vi "ZCR_IN_SIN_0_finder.vi"(10 "Noise amplitude":dbl format="%.2p", 11 "ZCR ON":waveform(dbl)[](array[waveform])=[{"t0"=timestamp(3707890383.8976955 s since 1904-01-01), "dt"=9.999999999999999e-05, "Y"=array[20000 elements], "attributes"=variant("NI_ChannelName"=variant(string "Tension_0"), "NI_UnitDescription"=variant(string "Volts"))}, {"t0"=timestamp(3707890383.8977456 s since 1904-01-01), "dt"=9.999999999999999e-05, "Y"=array[20000 elements], "attributes"=variant("NI_ChannelName"=variant(string "Tension_1"), "NI_UnitDescription"=variant(string "Volts"))}]) -> (3 "OFF SIN":i32[](array[numeric]))   [LabVIEW 2020, in "Library Commun.lvlib" / "Nodon_ZCR.lvclass"]
uses:
  Nodon_ZCR.lvclass
  <vilib>/Utility/miscctls.llb/LVRangeTypeDef.ctl
  <vilib>/measure/matone.llb/Extract Single Tone Information 1 Chan.vi
  Nodon_ZCR.lvclass/Nodon_ZCR.ctl
  <vilib>/measure/NI_MABase.lvlib
  <vilib>/measure/NI_MAPro.lvlib
panel:
  out "Waveform Graph 3":waveform(dbl)[](graph)
  in  "Point 2":i32
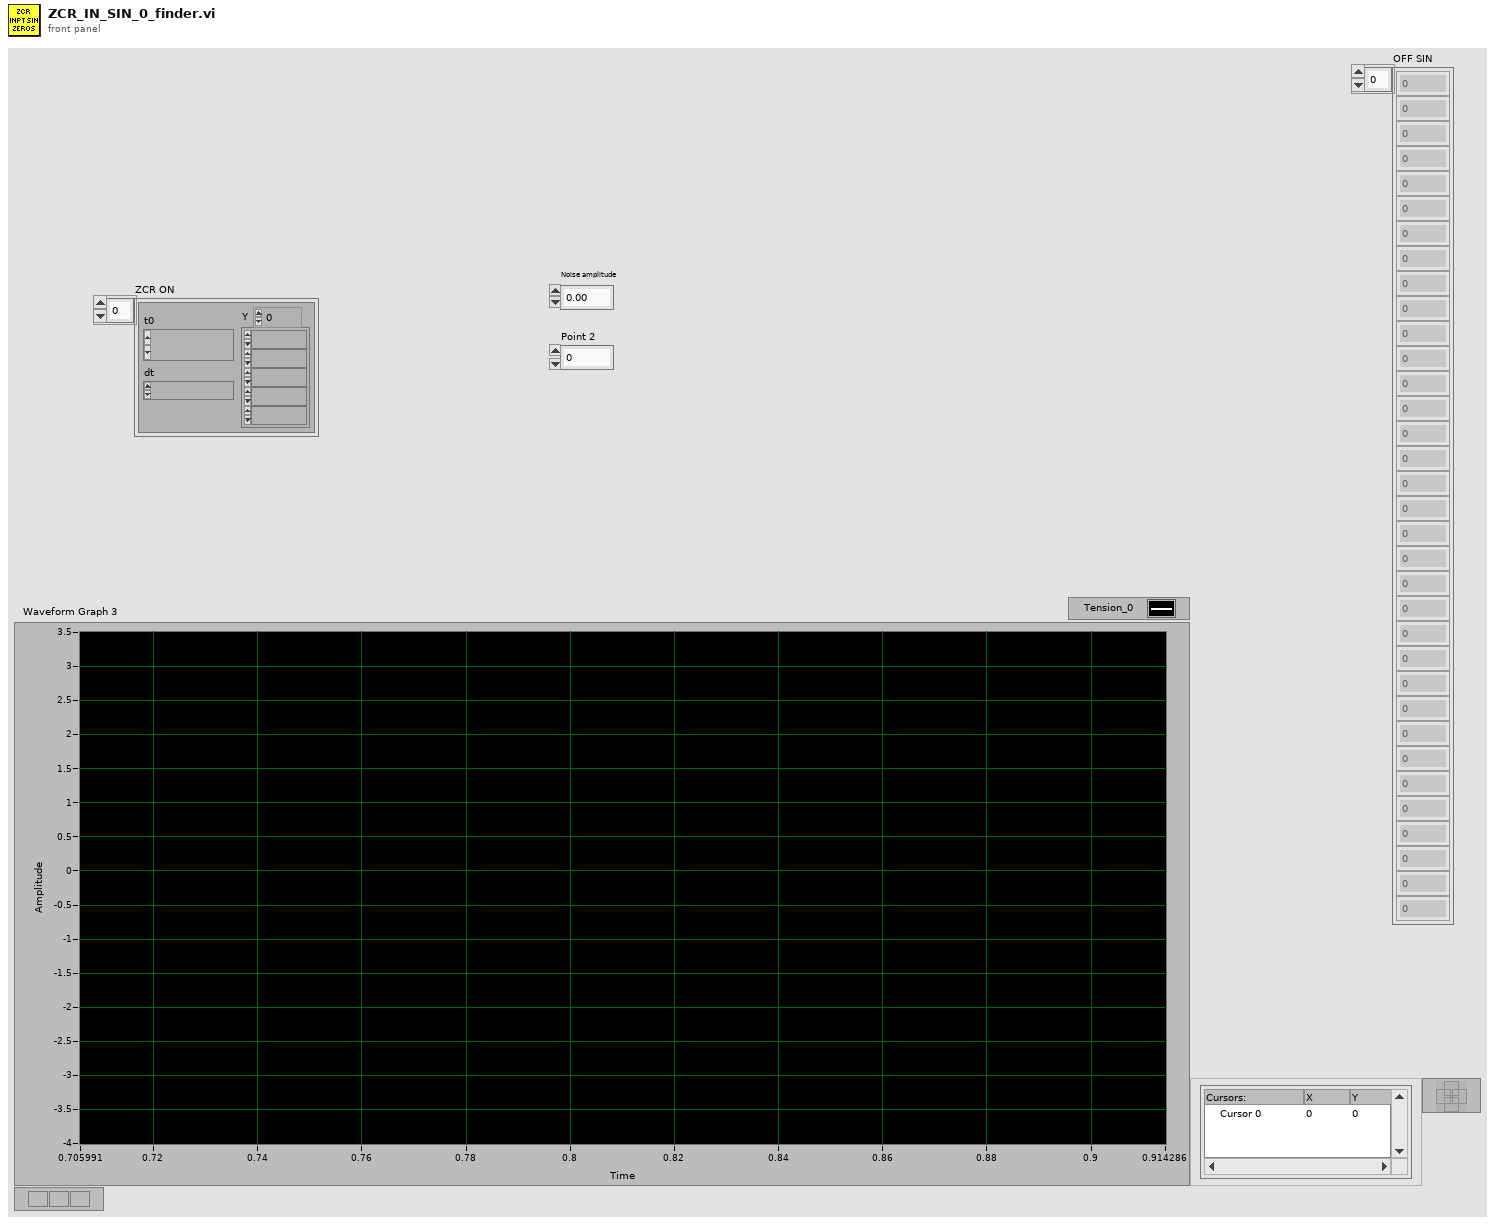
[diagram p1: front panel]
types:
  T1 = typedef "LVRangeTypeDef.ctl" = cluster{"Minimum":dbl, "Maximum":dbl, "Increment":dbl, "Minor Increment":dbl, "Start":dbl}
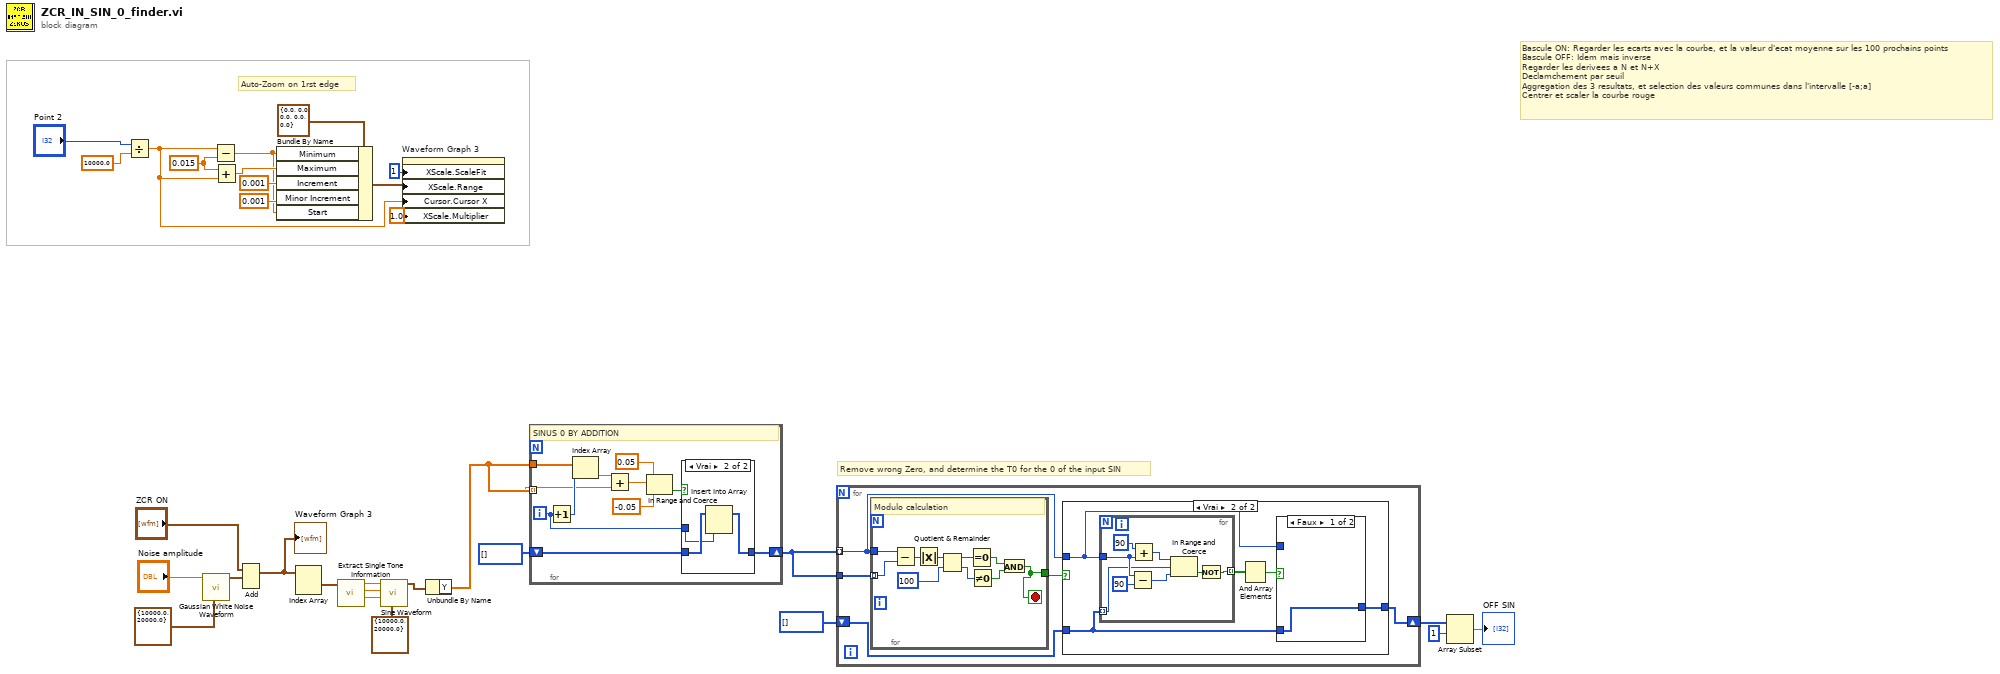
[diagram p0: block diagram]
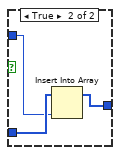
[diagram p3: hidden frame]
diagram:
  w20 = 0.015
  # "Bascule ON: Regarder les ecarts avec la courbe, et la valeur d'ecat moyenne sur les 100 prochains points\nBascule OFF: Idem mais inverse\nRegarder les derivees a N et N+X\nDeclamchement par seuil\nAggregation des 3 resultats, et selection des valeurs communes dans l'intervalle [-a;a]\nCentrer et scaler la courbe rouge"
  # "Remove wrong Zero, and determine the T0 for the 0 of the input SIN"
  # "Auto-Zoom on 1rst edge"
  n1 = Divide(x="Point 2", y=10000.0) -> (x/y=w11:dbl)
  n2 = call <vilib>:"Gaussian White Noise Waveform.vi"("sampling info"=cluster{"Fs":dbl, "#s":dbl} {"Fs"=10000.0, "#s"=20000.0}, "standard deviation"="Noise amplitude") -> ("signal out"=w27:waveform(dbl))  [unwired: 8 in, 1 out]
  n3 = Subtract(x=w11, y=w20) -> (x-y=w15:dbl)
  n4 = Add(x=w20, y=w11) -> (x+y=w18:dbl)
  n5 = Add(1:w27, 2:"ZCR ON") -> (0:w9:waveform(dbl)[])  [unwired: 1 in, 1 out]
  "Waveform Graph 3" <- w9
  n6 = Bundle By Name(cluster=T1 {"Minimum"=0.0, "Maximum"=0.0, "Increment"=0.0, "Minor Increment"=0.0, "Start"=0.0} ("X Scale.Range"), "Minimum"=w15, "Maximum"=w18, "Increment"=0.001, "Minor Increment"=0.001, "Start"=w15) -> (w14:T1)
  n7 = Index Array(array=w9) -> (element #1=w1:waveform(dbl))  [unwired: 2 in, 1 out]
  n8 = call-poly <vilib>:"Extract Single Tone Information.vi"("time signal in"=w1) -> ("detected phase (deg)"=w26:dbl, "detected amplitude"=w25:dbl, "detected frequency"=w24:dbl)  [unwired: 5 in, 3 out]
  n9 = call <vilib>:"Sine Waveform.vi"("sampling info"=cluster{"Fs":dbl, "#s":dbl} {"Fs"=10000.0, "#s"=20000.0}, "phase"=w26, "amplitude"=w25, "frequency"=w24) -> ("signal out"=w6:waveform(dbl))  [unwired: 6 in, 1 out]
  n10 = property on="Waveform Graph 3" class="GraphWF (strict)"("XScale.ScaleFit"=u8 1 ("X Scale.Scale Fit"), "XScale.Range"=w14, "Cursor.Cursor X"=w11, "XScale.Multiplier"=1.0 ("X Scale.Offset and Multiplier:Multiplier")) -> ()  [unwired: 2 in, 2 out]
  n11 = Unbundle By Name(w6) -> ("Y"=w5:dbl[])
  n12 = for {
    tunnel: w5 -> [w41]
    tunnel: w5 -> [w38] mode=indexing
    shift-right: [w36] -> w8
    shift-left: i32[] [] -> [w37]
    i -> [w35]
    # "SINUS 0 BY ADDITION"
    n13 = Increment(x=w35) -> (x+1=w40:i32)
    n14 = Index Array(array=w41, index=w40) -> (element=w39:dbl)
    n15 = Add(x=w39, y=w38) -> (x+y=w34:dbl)
    n16 = In Range and Coerce(upper limit=0.05 ("lower limit"), x=w34, lower limit=-0.05) -> (In Range?=w33:bool)  [unwired: 1 out]
    n17 = case shown="Vrai" w33 {
      tunnel: [w42 w44] -> w36
      tunnel: w37 -> [w42 w45]
      tunnel: w35 -> [_ w43]
      frame False {
      }
      frame True {
        n18 = Insert Into Array(array=w45, new element=w43) -> (w44:i32[])  [unwired: 1 in]
      }
    }
  }
  n19 = for {
    tunnel: w8 -> [w46] mode=indexing
    tunnel: w8 -> [w50]
    shift-right: [w47] -> w4
    shift-left: i32[] [] -> [w48]
    n20 = for {
      tunnel: w46 -> [w78]
      tunnel: w50 -> [w77] mode=indexing
      tunnel: [w69] -> w49
      stop <- w69 stop-if-true
      # "Modulo calculation"
      n21 = Subtract(x=w78, y=w77) -> (x-y=w76:i32)
      n22 = Absolute Value(x=w76) -> (abs(x)=w75:i32)
      n23 = Quotient & Remainder(x=w75, y=100) -> (x-y*floor(x/y)=w73:i32, floor(x/y)=w72:i32)
      n24 = Equal To 0?(x=w73) -> (x = 0?=w71:bool)
      n25 = Not Equal To 0?(x=w72) -> (x != 0?=w70:bool)
      n26 = And(x=w71, y=w70) -> (x .and. y?=w69:bool)
    }
    n27 = case shown="Vrai" w49 {
      tunnel: w48 -> [w51 w54]
      tunnel: [w51 w53] -> w47
      tunnel: w46 -> [_ w52]
      frame False {
      }
      frame True {
        n28 = for {
          tunnel: w52 -> [w64]
          tunnel: w54 -> [w61] mode=indexing
          tunnel: [w62] -> w56 mode=indexing
          n29 = Subtract(x=w64, y=90) -> (x-y=w65:i32)
          n30 = Add(x=90, y=w64) -> (x+y=w66:i32)
          n31 = In Range and Coerce(upper limit=w66, x=w61, lower limit=w65) -> (In Range?=w63:bool)  [unwired: 1 out]
          n32 = Not(x=w63) -> (.not. x?=w62:bool)
        }
        n33 = And Array Elements(Boolean array=w56) -> (logical AND=w55:bool)
        n34 = case shown="Faux" w55 {
          tunnel: w54 -> [w57 w59]
          tunnel: [w57 w60] -> w53
          tunnel: w52 -> [_ w58]
          frame False {
          }
          frame True {
            n35 = Insert Into Array(array=w59, new element=w58) -> (w60:i32[])  [unwired: 1 in]
          }
        }
      }
    }
  }
  n36 = Array Subset(array=w4, index=1) -> (→"OFF SIN":i32[])  [unwired: 1 in]
